vi "get_pico_data.vi"(8 "error in":errorcluster, 11 "PicoScope Acquisition Settings":T1={"Channel A Settings"={"Enabled"=TRUE, "Coupling"=1, "Range"=6, "Analogue Offset"=0.0}, "Channel B Settings"={"Enabled"=TRUE, "Coupling"=1, "Range"=6, "Analogue Offset"=0.0}, "Trigger Options"={"Trigger Enabled"=FALSE, "Trigger Source"=enum."Channel A", "Trigger Threshold (-5 to 5 V)"=0.0, "Trigger Slope"=2, "Trigger Delay (ms)"=0.0, "Auto Trigger Time (ms)"=1000}, "Pico Scope Inititalization Settings"={"USB Power"=FALSE, "Use Serial Number"=FALSE, "Resolution"=0, "Serial Number"="", "Handle"=0}, "Use PicoScope?"=FALSE, "Acquisition Settings"={"Pre Trigger Time (s)"=512.0, "Post Trigger Time (s)"=512.0, "Resolution (s)"=34.36, "Down-Sample Mode"=0, "Down Sample Ratio"=1, "Four Channel Device"=FALSE}} {"Acquisition Settings"."Down Sample Ratio" min=1 step=1; "Acquisition Settings"."Down-Sample Mode" items=["None"=0, "Aggregate"=1, "Decimate"=2, "Average"=4]; "Acquisition Settings"."Resolution (s)" min=8e-09 max=34.36 step=8e-09 format="%#_6p"; "Acquisition Settings"."Post Trigger Time (s)" min=0.0 format="%#_6p"; "Acquisition Settings"."Pre Trigger Time (s)" min=0.0 format="%#_6p"; "Pico Scope Inititalization Settings"."Resolution" items=["8-bit", "12-bit", "14-bit", "15-bit (max. 2 ch.)", "16-bit (max. 1 ch.)"]; "Trigger Options"."Trigger Slope" items=["Rising"=2, "Falling"=3]; "Channel B Settings"."Range" items=["10 mV", "20 mV", "50 mV", "100 mV", "200 mV", "500 mV", "1 V", "2 V", "5 V", "10 V", "20 V", "50 V ", "100 V"]; "Channel B Settings"."Coupling" items=["AC", "DC"]; "Channel A Settings"."Range" items=["10 mV", "20 mV", "50 mV", "100 mV", "200 mV", "500 mV", "1 V", "2 V", "5 V", "10 V", "20 V", "50 V ", "100 V"]; "Channel A Settings"."Coupling" items=["AC", "DC"]}) -> (0 "error out":errorcluster, 2 "Channel B Out":dbl[][](array[numeric]), 3 "Channel A Out":dbl[][](array[numeric]))   [LabVIEW 2013]
uses:
  Controls/PicoScope/pico_control_panel.ctl
  Controls/PicoScope/pico_channel_settings.ctl
  Controls/PicoScope/pico_trigger.ctl
  Controls/PicoScope/pico_init_settings.ctl
panel:
  out "Channel B Buffer":i16[](array[numeric])
  out "Channel A Buffer":i16[](array[numeric])
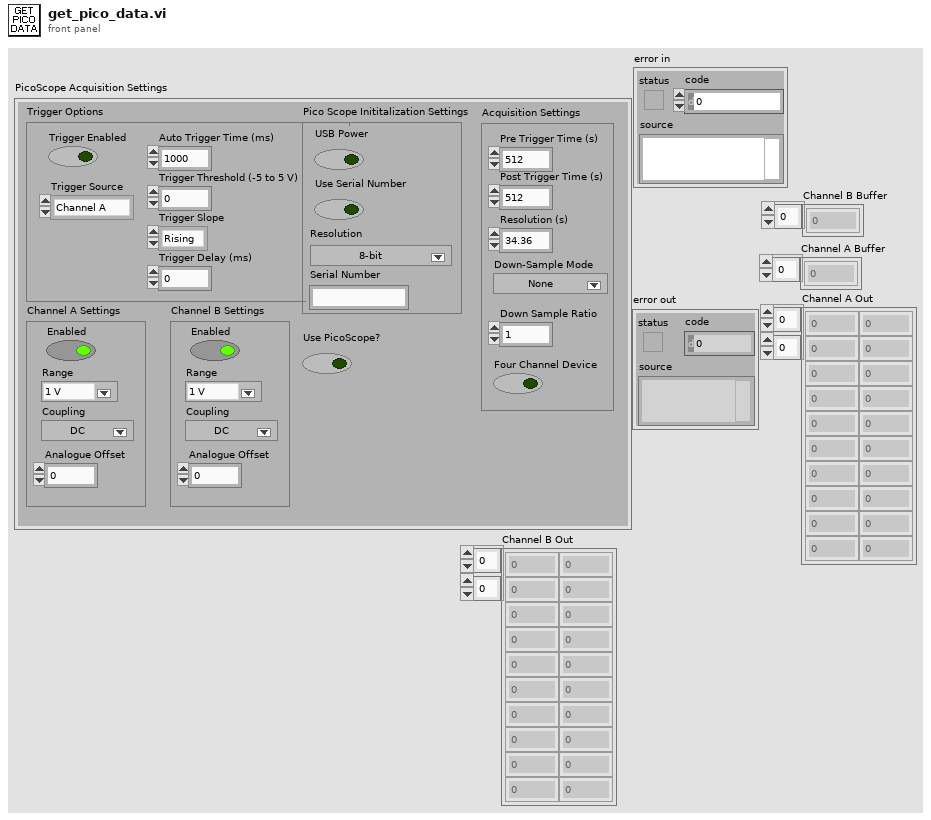
[diagram p1: front panel]
types:
  T1 = typedef "pico_control_panel.ctl" = cluster{"Channel A Settings":T2, "Channel B Settings":T2, "Trigger Options":T3, "Pico Scope Inititalization Settings":T4, "Use PicoScope?":bool, "Acquisition Settings":cluster{"Pre Trigger Time (s)":dbl, "Post Trigger Time (s)":dbl, "Resolution (s)":dbl, "Down-Sample Mode":i32, "Down Sample Ratio":u32, "Four Channel Device":bool}}
  T2 = typedef "pico_channel_settings.ctl" = cluster{"Enabled":bool, "Coupling":i16, "Range":u16, "Analogue Offset":sgl}
  T3 = typedef "pico_trigger.ctl" = cluster{"Trigger Enabled":bool, "Trigger Source":enum16{"Channel A", "Channel B", "Channel C", "Channel D", "Ext."}, "Trigger Threshold (-5 to 5 V)":dbl, "Trigger Slope":u16, "Trigger Delay (ms)":dbl, "Auto Trigger Time (ms)":i16}
  T4 = typedef "pico_init_settings.ctl" = cluster{"USB Power":bool, "Use Serial Number":bool, "Resolution":i32, "Serial Number":string, "Handle":i16}
  T5 = cluster{"Pre Trigger Time (s)":dbl, "Post Trigger Time (s)":dbl, "Resolution (s)":dbl, "Down-Sample Mode":i32, "Down Sample Ratio":u32, "Four Channel Device":bool}
  T6 = cluster{"preTriggerSamples":u32, "postTriggerSamples":u32, "timebase":u32, "Down-Sample Mode":i32, "Down Sample Ratio":u32, "Four Channel Device":bool}
  T7 = cluster{"Channel D Buffer":i16[], "Channel C Buffer":i16[], "Channel B Buffer":i16[], "Channel A Buffer":i16[]}
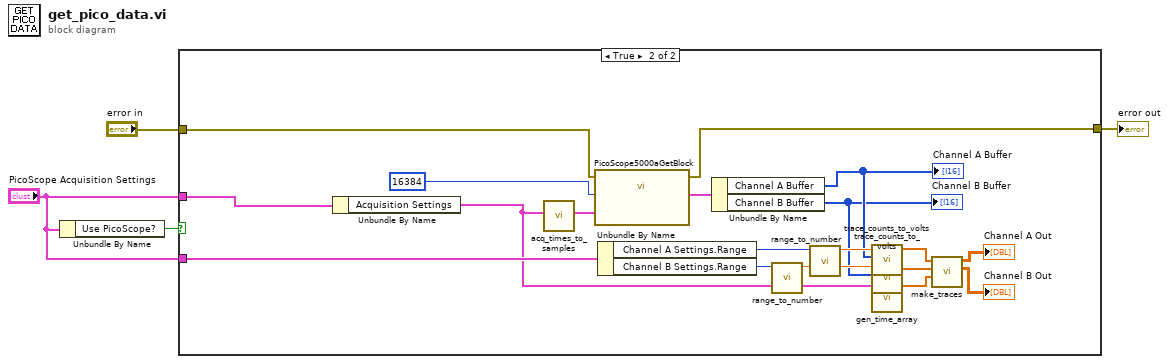
[diagram p0: block diagram]
diagram:
  n1 = Unbundle By Name("PicoScope Acquisition Settings") -> ("Use PicoScope?"=w2:bool)
  n2 = case shown="True" w2 {
    tunnel: "PicoScope Acquisition Settings" -> [_ w24]
    tunnel: "error in" -> [w5 w23]
    tunnel: [w5 w20] -> w3
    tunnel: "PicoScope Acquisition Settings" -> [_ w19]
    frame False {
    }
    frame True {
      n3 = Unbundle By Name(w24) -> ("Acquisition Settings"=w12:T5)
      n4 = call "acq_times_to_samples.vi"("Acquisition Settings"=w12) -> ("Settings to Pico"=w22:T6)  [unwired: 10 in]
      n5 = call "PicoScope5000aGetBlock.vi"("error in"=w23, "handle in"=i16 16384, "Acquisition Settings"=w22) -> ("error out"=w20:errorcluster, "Buffers (Max or non-aggregated)"=w21:T7)  [unwired: 3 in, 3 out]
      n6 = Unbundle By Name(w19) -> ("Channel A Settings.Range"=w17:u16, "Channel B Settings.Range"=w18:u16)
      n7 = Unbundle By Name(w21) -> ("Channel A Buffer"=w15:i16[], "Channel B Buffer"=w13:i16[])
      "Channel A Buffer" <- w15
      "Channel B Buffer" <- w13
      n8 = call "range_to_number.vi"("Channel A Settings.Range"=w18) -> ("Voltage Range"=w14:dbl)  [unwired: 10 in]
      n9 = call "range_to_number.vi"("Channel A Settings.Range"=w17) -> ("Voltage Range"=w16:dbl)  [unwired: 10 in]
      n10 = call "trace_counts_to_volts.vi"("Counts In"=w15, "Voltage Range"=w16) -> ("Voltage Out"=w10:dbl[])  [unwired: 9 in]
      n11 = call "trace_counts_to_volts.vi"("Counts In"=w13, "Voltage Range"=w14) -> ("Voltage Out"=w11:dbl[])  [unwired: 9 in]
      n12 = call "gen_time_array.vi"("Acquisition Settings"=w12) -> ("Time Out"=w9:dbl[])  [unwired: 10 in]
      n13 = call "make_traces.vi"("Time"=w9, "Channel B"=w11, "Channel A"=w10) -> ("Channel B Out"=→"Channel B Out":dbl[][], "Channel A Out"=→"Channel A Out":dbl[][])  [unwired: 7 in]
    }
  }
  "error out" <- w3
